vi "calculate_slider_locations.vi"(8 "error in":errorcluster, 11 "Docked? (F)":bool) -> (0 "error out":errorcluster, 2 "sliding_panel_right_coord":i32, 3 "sliding_panel_left_coord":i32)   [LabVIEW 2018]
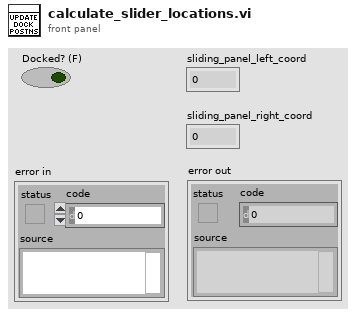
[diagram p1: front panel]
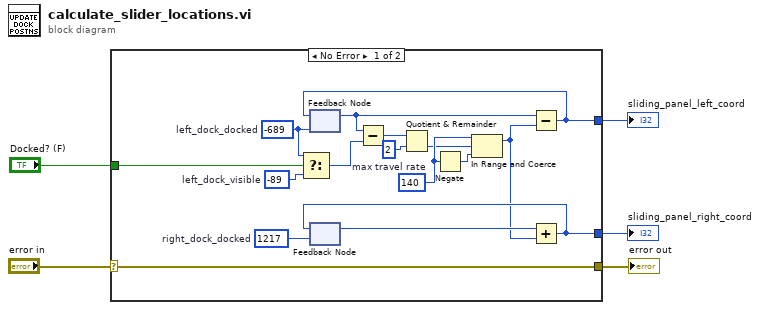
[diagram p0: block diagram]
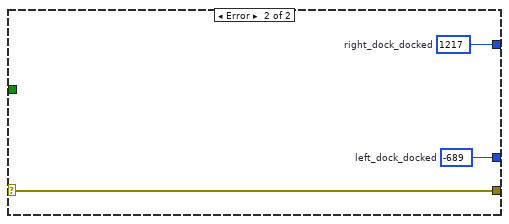
[diagram p2: hidden frame]
diagram:
  n1 = case shown="No Error" "error in" {
    selector: "error in" -> [w8 w24]
    tunnel: "Docked? (F)" -> [w20 _]
    tunnel: [w16 w22] -> w4
    tunnel: [w14 w23] -> w3
    tunnel: [w8 w24] -> w1
    frame No Error {
      w21 = 140  # max travel rate
      w18 = -89  # left_dock_visible
      w17 = 1217  # right_dock_docked
      w6 = -689  # left_dock_docked
      n2 = Select(t=w6, s=w20, f=w18) -> (s? t:f=w19:i32)
      n3 = feedback #1(w6) -> (w13:i32)
      n4 = feedback #2(w17) -> (w15:i32)
      n5 = Subtract(x=w13, y=w19) -> (x-y=w11:i32)
      n6 = Quotient & Remainder(x=w11, y=2) -> (floor(x/y)=w10:i32)  [unwired: 1 out]
      n7 = Negate(x=w21) -> (-x=w12:i32)
      n8 = In Range and Coerce(upper limit=w21, x=w10, lower limit=w12) -> (coerced(x)=w7:i32)  [unwired: 1 out]
      n9 = Subtract(x=w13, y=w7) -> (x-y=w14:i32)
      n10 = feedback-in #1(w14) -> ()
      n11 = Add(x=w15, y=w7) -> (x+y=w16:i32)
      n12 = feedback-in #2(w16) -> ()
    }
    frame Error {
      w22 = -689  # left_dock_docked
      w23 = 1217  # right_dock_docked
    }
  }
  "sliding_panel_right_coord" <- w4
  "sliding_panel_left_coord" <- w3
  "error out" <- w1
